vi "WPI_UltrasonicOpen.vi"   [LabVIEW 2017]
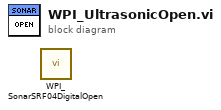
[diagram p0: block diagram]
diagram:
  n1 = call <vilib>:"WPI_SonarSRF04DigitalOpen.vi"() -> ()  [unwired: 10 in, 2 out]
